vi "DiscoverCamNames.vi"(10 "Rescan":bool, 11 "PicturesPath":path) -> (1 "CamNames":string[](array[string]))   [LabVIEW 2022 SP3]
uses:
  <vilib>/Utility/config.llb/NI_LVConfig.lvlib
  <vilib>/Utility/config.llb/Write Key (String).vi
panel:
  # "Looks for CamNames.ini and uses if found. If not found, or Rescan pressed, scans folder, and creates CamNames.ini\nWebcamReadandOverlay now creates CamNames.ini as it runs.\nTCRL 2024-06-21\n\nNow looks for WebcamsNew.ini and uses if present\nTCRL 2024-06-18\n\nTook 1900s to complete on folder of XXX files\nFreezes LV completely while scanning\nNeeds something doing! TCRL 2022-01-18"
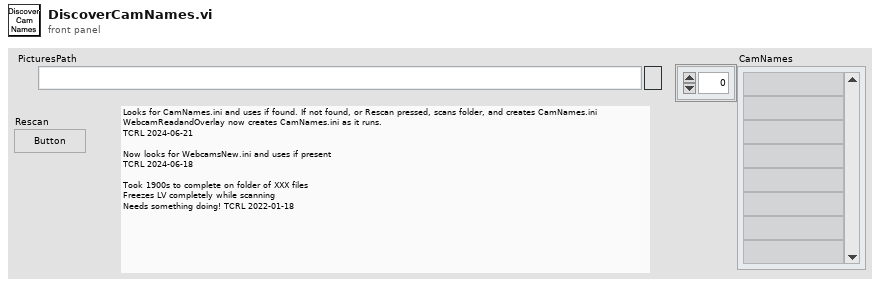
[diagram p1: front panel]
types:
  T1 = typedef "NI_LVConfig.lvlib/Config Data RefNum.ctl" = refnum<k1>
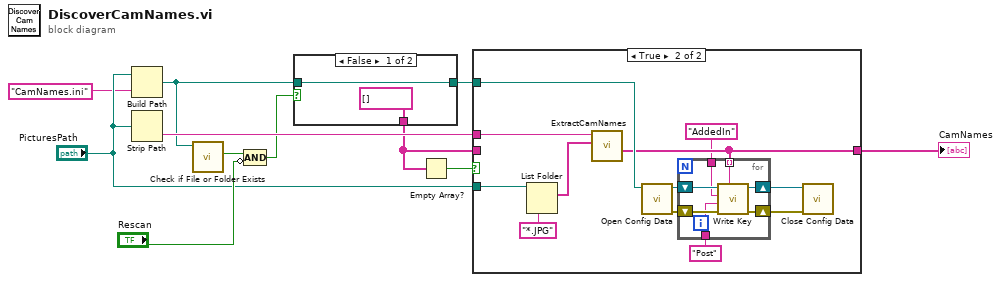
[diagram p0: block diagram]
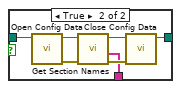
[diagram p2: hidden frame]
diagram:
  n1 = Build Path(base path="PicturesPath", name or relative path="CamNames.ini") -> (appended path=w6:path)
  n2 = Strip Path(path="PicturesPath") -> (name=w7:string)  [unwired: 1 out]
  n3 = call <vilib>:"Check if File or Folder Exists.vi"("path"=w6) -> ("file or folder exists?"=w1:bool)  [unwired: 8 in, 2 out]
  n4 = Compound Arithmetic op=AND(w1, invert "Rescan") -> (w2:bool)
  n5 = case shown="False" w2 {
    tunnel: [string[] [] ("section names") w16] -> w4
    tunnel: w6 -> [w12 w15]
    tunnel: [w12 w14] -> w3
    frame False {
    }
    frame True {
      n6 = call <vilib>:"Open Config Data.vi"("configuration file path"=w15) -> ("error out"=w20:errorcluster, "refnum"=w19:T1)  [unwired: 8 in, 1 out]
      n7 = call <vilib>:"Get Section Names.vi"("error in (no error)"=w20, "refnum"=w19) -> ("error out"=w18:errorcluster, "section names"=w16:string[], "refnum out"=w17:T1)  [unwired: 7 in]
      n8 = call <vilib>:"Close Config Data.vi"("error in (no error)"=w18, "refnum"=w17) -> ("file path"=w14:path)  [unwired: 8 in, 1 out]
    }
  }
  n9 = Empty Array?(array=w4) -> (empty?=w5:bool)
  n10 = case shown="True" w5 {
    tunnel: w7 -> [_ w32]
    tunnel: [w21 w25] -> w11
    tunnel: "PicturesPath" -> [_ w31]
    tunnel: w4 -> [w21 _]
    tunnel: w3 -> [_ w28]
    frame False {
    }
    frame True {
      n11 = List Folder(path=w31, pattern="*.JPG") -> (filenames=w33:string[])  [unwired: 2 in, 3 out]
      n12 = call "ExtractCamNames.vi"("filenames"=w33, "name"=w32) -> ("CamNames"=w25:string[])  [unwired: 9 in]
      n13 = call <vilib>:"Open Config Data.vi"("configuration file path"=w28) -> ("error out"=w27:errorcluster, "refnum"=w29:T1)  [unwired: 8 in, 1 out]
      n14 = for {
        shift-right: [w40] -> w30
        shift-left: w29 -> [w39]
        shift-right: [w37] -> w26
        shift-left: w27 -> [w38]
        tunnel: w25 -> [w36] mode=indexing
        tunnel: "AddedIn" ("key") -> [w35]
        tunnel: "Post" ("key") -> [w34]
        n15 = call-poly <vilib>:"Write Key.vi"("section"=w36, "error in (no error)"=w38, "value"=w34, "key"=w35, "refnum"=w39) -> ("error out"=w37:errorcluster, "refnum out"=w40:T1)  [unwired: 4 in, 1 out]
      }
      n16 = call <vilib>:"Close Config Data.vi"("error in (no error)"=w26, "refnum"=w30) -> ()  [unwired: 8 in, 2 out]
    }
  }
  "CamNames" <- w11
